vi "String2StringArray.vi"(1 "String":string) -> (0 "Array of Char":string[](array[string]))   [LabVIEW 2020]
doc: "converts string to array of char"
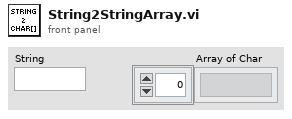
[diagram p1: front panel]
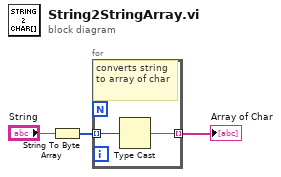
[diagram p0: block diagram]
diagram:
  n1 = String To Byte Array(string="String") -> (unsigned byte array=w3:u8[])
  n2 = for {
    tunnel: [w5] -> w2 mode=indexing
    tunnel: w3 -> [w4] mode=indexing
    # "converts string to array of char"
    n3 = Type Cast(x=w4) -> (*(type *) &x=w5:string)  [unwired: 1 in]
  }
  "Array of Char" <- w2
